vi "Channel_CreateChannel.vi"(6 "Data Reference":T1 format="%.0x", 7 "Meta Data":T2[](array[typedef]), 8 "error in (no error)":errorcluster, 9 "Decimation":i32, 10 "Wfm?":bool, 11 "Name":string) -> (0 "error out":errorcluster, 3 "Channel out":refnum<class "Channel.lvclass">)   [LabVIEW 2023, in "Channel.lvclass"]
doc: "Create a new channel class object based on the given input details."
uses:
  Channel.lvclass
  Meta Data.ctl
  <vilib>/NI VeriStand/Custom Device API/Data Reference.ctl
  Channel.lvclass/Channel.ctl
  <vilib>/NI VeriStand/Custom Device API/Custom Device API.lvlib
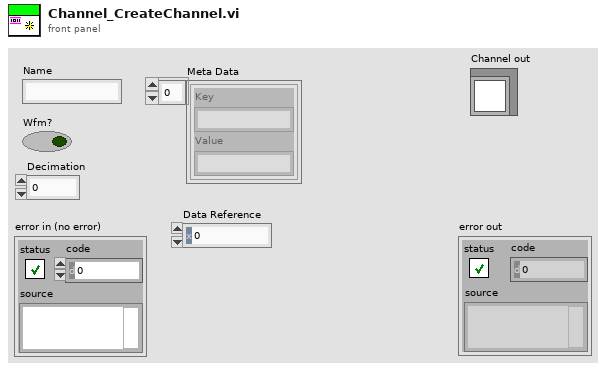
[diagram p1: front panel]
types:
  T1 = typedef "Custom Device API.lvlib/Data Reference.ctl" = i32
  T2 = typedef "Meta Data.ctl" = cluster{"Key":string, "Value":string}
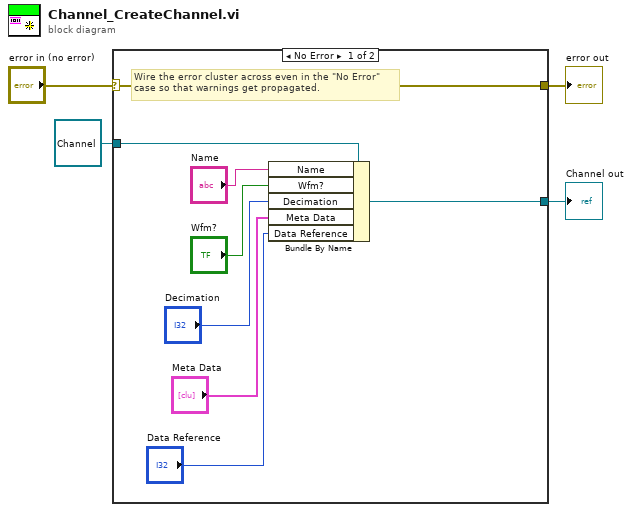
[diagram p0: block diagram]
diagram:
  n1 = case shown="No Error" "error in (no error)" {
    selector: "error in (no error)" -> [w12 w14]
    tunnel: [w12 w14] -> w3
    tunnel: refnum<class "Channel.lvclass"> refnum ("Channel.lvclass") -> [w11 w13]
    tunnel: [w10 w13] -> w1
    frame No Error {
      # "Wire the error cluster across even in the \"No Error\"\ncase so that warnings get propagated."
      n2 = Bundle By Name(cluster=w11, "Name"="Name", "Wfm?"="Wfm?", "Decimation"="Decimation", "Meta Data"="Meta Data", "Data Reference"="Data Reference") -> (w10:refnum<class "Channel.lvclass">)
    }
    frame Error {
    }
  }
  "error out" <- w3
  "Channel out" <- w1
